vi "Read Range.vi"(0 "VISA resource name":refnum<visa-resource-name>="COM1", 5 "Address (00)":i32 format="%02.0f", 11 "error in (no error)":errorcluster) -> (4 "VISA resource name out":refnum<visa-resource-name>, 6 "Target Units":string, 8 "Flow Rate Units":string, 10 "Pump status":T1 items=["Error - Can't read status"=-1, "Stopped"=0, "Infusing"=1, "Withdrawing"=2, "Pump stalled"=3, "Stopped at infuse limit"=4, "Stopped at withdraw limit"=5, "Emergency stop"=6, "Stopped at target volume"=7], 15 "error out":errorcluster)   [LabVIEW 2015]
doc: "This VI returns the range message.\nThe range message corresponds to the units set in the Configure Flow Rate.vi\n\nModified from original which is Copyright 2005, National Instruments Corporation.\n\nModifications Copyright 2009, Jeff Gelles, Brandeis University"
uses:
  Pump status.ctl
panel:
  out "Number of tries to get units":i32
  out "Output String":string
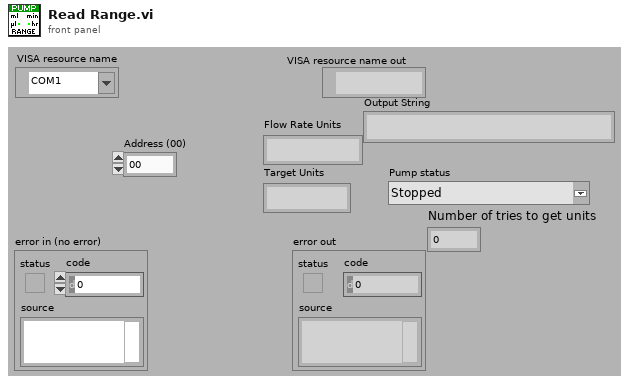
[diagram p1: front panel]
types:
  T1 = typedef "Pump status.ctl" = i8
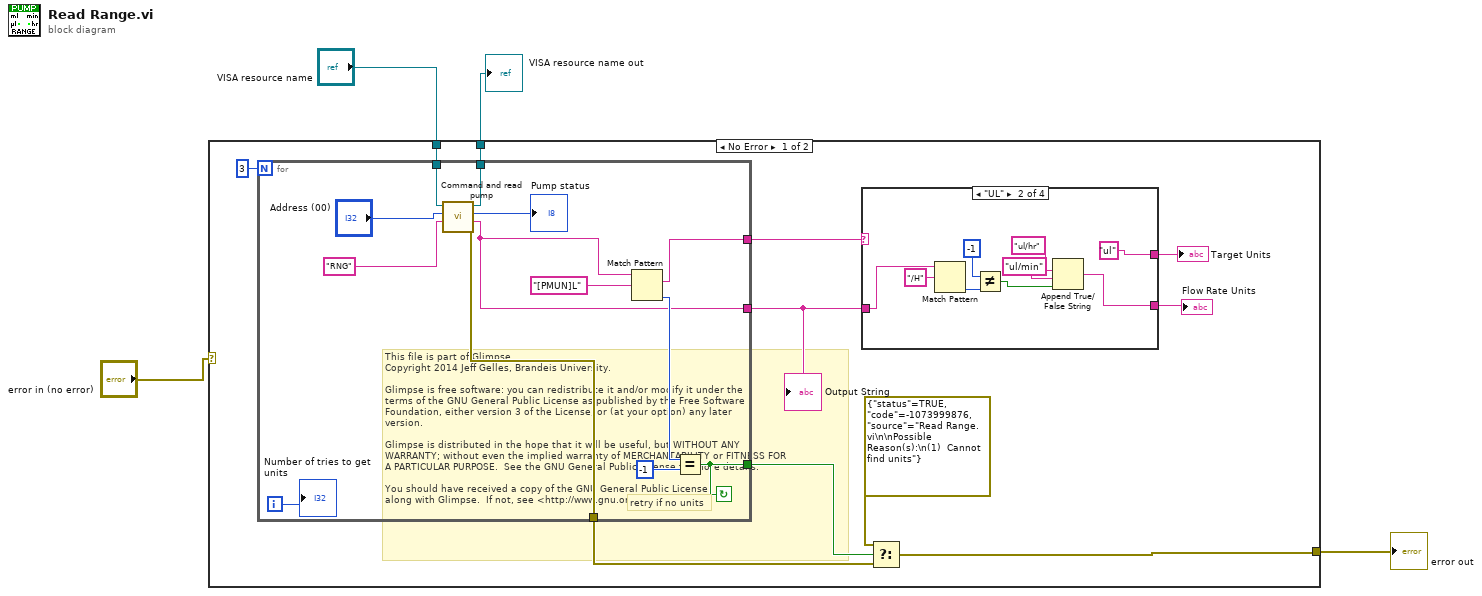
[diagram p0: block diagram]
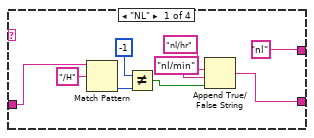
[diagram p2: hidden frame]
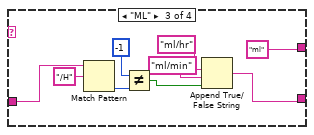
[diagram p3: hidden frame]
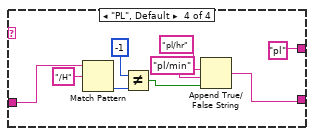
[diagram p4: hidden frame]
diagram:
  # "This file is part of Glimpse. \nCopyright 2014 Jeff Gelles, Brandeis University.    \n\nGlimpse is free software: you can redistribute it and/or modify it under the \nterms of the GNU General Public License as published by the Free Software \nFoundation, either version 3 of the License, or (at your option) any later \nversion.\n\nGlimpse is distributed in the hope that it will be useful, but WITHOUT ANY \nWARRANTY; without even the implied warranty of MERCHANTABILITY or FITNESS FOR \nA PARTICULAR PURPOSE.  See the GNU General Public License for more details.\n\nYou should have received a copy of the GNU General Public License\nalong with Glimpse.  If not, see <http://www.gnu.org/licenses/>."
  n1 = case shown="No Error" "error in (no error)" {
    selector: "error in (no error)" -> [_ w65]
    tunnel: [w12 w65] -> w4
    tunnel: [w7 w66] -> w3
    tunnel: "VISA resource name" -> [w6 w66]
    frame No Error {
      n2 = for {
        N: 3 -> [_]
        tunnel: [w17] -> w13
        tunnel: [w26] -> w10
        tunnel: [w23] -> w9
        tunnel: [w22] -> w8
        tunnel: [w21] -> w7
        tunnel: w6 -> [w18]
        i -> [w16]
        stop <- w17 continue-if-true
        # "retry if no units"
        n3 = call "Command and read pump.vi"("command"="RNG", "Address (00)"="Address (00)", "VISA resource name"=w18) -> ("error out"=w22:errorcluster, "Output String"=w23:string, "Pump status"=→"Pump status":T1, "VISA resource name out"=w21:refnum<visa-resource-name>)  [unwired: 1 in, 4 out]
        n4 = Match Pattern(string=w23, regular expression="[PMUN]L") -> (match substring=w26:string, offset past match=w25:i32)  [unwired: 3 out]
        n5 = Equal?(x=w25, y=-1 ("x")) -> (x = y?=w17:bool)
        "Number of tries to get units" <- w16
      }
      "Output String" <- w9
      n6 = case shown="\"UL\"" w10 {
        tunnel: w9 -> [w31 w40 w47 w56]
        tunnel: ["nl" ("Target Units") "ul" ("Target Units") "ml" ("Target Units") "pl" ("Target Units")] -> w15
        tunnel: [w30 w39 w48 w57] -> w14
        frame "NL" {
          n7 = Match Pattern(string=w31, regular expression="/H") -> (offset past match=w34:i32)  [unwired: 4 out]
          n8 = Not Equal?(x=-1, y=w34) -> (x != y?=w32:bool)
          n9 = Append True/False String(1:w32, 2:"nl/min" ("true string"), 3:"nl/hr" ("true string")) -> (0:w30:string)  [unwired: 1 out]
        }
        frame "UL" {
          n10 = Match Pattern(string=w40, regular expression="/H") -> (offset past match=w43:i32)  [unwired: 4 out]
          n11 = Not Equal?(x=-1, y=w43) -> (x != y?=w41:bool)
          n12 = Append True/False String(1:w41, 2:"ul/min" ("true string"), 3:"ul/hr" ("true string")) -> (0:w39:string)  [unwired: 1 out]
        }
        frame "ML" {
          n13 = Match Pattern(string=w47, regular expression="/H") -> (offset past match=w52:i32)  [unwired: 4 out]
          n14 = Not Equal?(x=-1, y=w52) -> (x != y?=w50:bool)
          n15 = Append True/False String(1:w50, 2:"ml/min" ("true string"), 3:"ml/hr" ("true string")) -> (0:w48:string)  [unwired: 1 out]
        }
        frame "PL", Default {
          n16 = Match Pattern(string=w56, regular expression="/H") -> (offset past match=w60:i32)  [unwired: 4 out]
          n17 = Not Equal?(x=-1, y=w60) -> (x != y?=w58:bool)
          n18 = Append True/False String(1:w58, 2:"pl/min" ("true string"), 3:"pl/hr" ("true string")) -> (0:w57:string)  [unwired: 1 out]
        }
      }
      "Target Units" <- w15
      "Flow Rate Units" <- w14
      n19 = Select(t=errorcluster {"status"=TRUE, "code"=-1073999876, "source"="Read Range.vi\n\nPossible Reason(s):\n(1)  Cannot find units"}, s=w13, f=w8) -> (s? t:f=w12:errorcluster)
    }
    frame Error {
    }
  }
  "VISA resource name out" <- w3
  "error out" <- w4
